vi "Set TimeToPlot.vi"(8 "error in (no error)":errorcluster, 10 "Time to Plot":dbl=1800.0 format="%<%H:%M:%S>t", 11 "Loop data in":T1 {"PanelMap"."Data"."Plot Bounds (%)"."Bottom (%)" format="%.2f"; "PanelMap"."Data"."Plot Bounds (%)"."Top (%)" format="%.2f"; "PanelMap"."Data"."Plot Bounds (%)"."Right (%)" format="%.2f"; "PanelMap"."Data"."Plot Bounds (%)"."Left (%)" format="%.2f"}) -> (0 "error out":errorcluster, 3 "Loop data out":T1 {"PanelMap"."Data"."Plot Bounds (%)"."Bottom (%)" format="%.2f"; "PanelMap"."Data"."Plot Bounds (%)"."Top (%)" format="%.2f"; "PanelMap"."Data"."Plot Bounds (%)"."Right (%)" format="%.2f"; "PanelMap"."Data"."Plot Bounds (%)"."Left (%)" format="%.2f"})   [LabVIEW 2021, in "MultiRocketPlotPanel.lvclass"]
uses:
  Classes/MultiPlotPanel/MultiRocketPlotPanel.lvclass
  Loop Data.ctl
  <vilib>/IlluminatedG/IG OOPanel/OOPanel/Manager/Manager.lvclass
  Panel Map.ctl
  Panel Map Data.ctl
  <userlib>/bjustice/RocketPlot/Classes/RocketPlotPanel/RocketPlotPanel.lvclass
  Window Position.ctl
  <vilib>/IlluminatedG/IG OOPanel/OOPanel/Panel/Panel Events.ctl
  <vilib>/IlluminatedG/IG OOPanel/OOPanel/Panel/Visbility Event Data.ctl
  <vilib>/IlluminatedG/IG OOPanel/OOPanel/Visibility State.ctl
  <vilib>/IlluminatedG/IG OOPanel/OOPanel/Close Reason.ctl
  <userlib>/bjustice/RocketPlot/Classes/RocketPlotPanel/RocketPlotPanel.lvclass/RocketPlotPanel.ctl
  <userlib>/bjustice/RocketPlot/Classes/RocketPlotPanel/Read RocketPlotHandle.vi
  <userlib>/bjustice/RocketPlot/Classes/RocketPlotHandle/RocketPlotHandle.lvclass
  <vilib>/IlluminatedG/IG OOPanel/OOPanel/OOPanel.lvlib
  <vilib>/IlluminatedG/IG OOPanel/OOPanel/Panel/Panel.lvclass
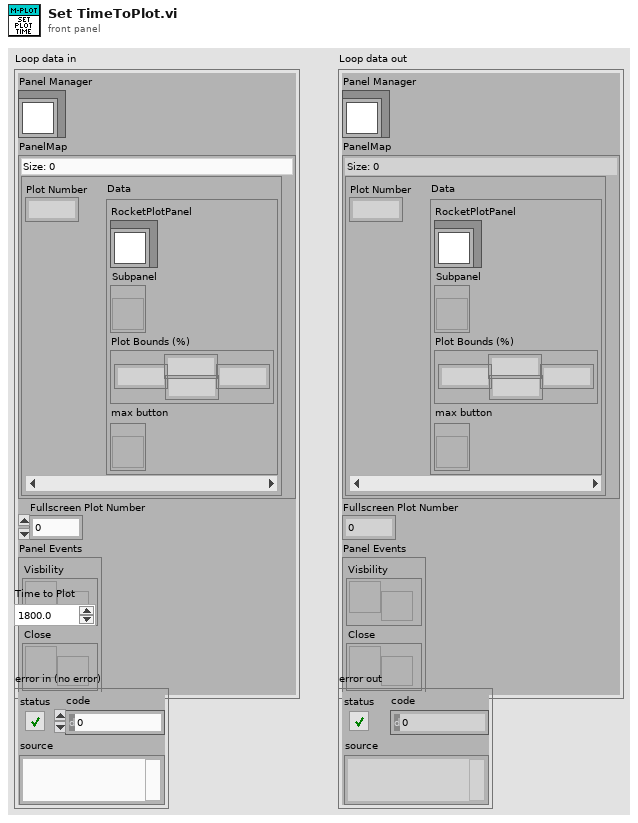
[diagram p1: front panel]
types:
  T1 = typedef "MultiRocketPlotPanel.lvclass/Loop Data.ctl" = cluster{"Panel Manager":refnum<class "Manager.lvclass">, "PanelMap":T2, "Fullscreen Plot Number":i32, "Panel Events":T5}
  T2 = typedef "MultiRocketPlotPanel.lvclass/Panel Map.ctl" = map{i32, T3}
  T3 = typedef "MultiRocketPlotPanel.lvclass/Panel Map Data.ctl" = cluster{"RocketPlotPanel":refnum<class "RocketPlotPanel.lvclass">, "Subpanel":refnum<vi>, "Plot Bounds (%)":T4, "max button":refnum<vi>}
  T4 = typedef "MultiRocketPlotPanel.lvclass/Window Position.ctl" = cluster{"Left (%)":dbl, "Top (%)":dbl, "Right (%)":dbl, "Bottom (%)":dbl}
  T5 = typedef "OOPanel.lvlib/Panel.lvclass/Panel Events.ctl" = cluster{"Visbility":refnum<user-event>, "Close":refnum<user-event>}
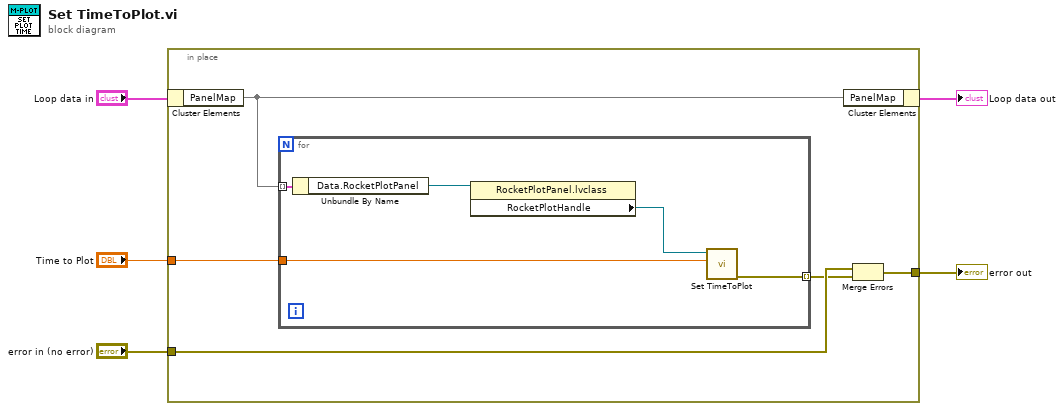
[diagram p0: block diagram]
diagram:
  n1 = in-place {
    in-place-border: "error in (no error)" -> [w9]
    in-place-border: [w6] -> w2
    in-place-border: "Time to Plot" -> [w7]
    n2 = in-place-cluster #1("Loop data in") -> ("PanelMap"=w10:T2)
    n3 = for {
      tunnel: w10 -> [w15] mode=indexing
      tunnel: [w11] -> w8 mode=indexing
      tunnel: w7 -> [w12]
      n4 = Unbundle By Name(w15) -> ("Data.RocketPlotPanel"=w14:refnum<class "RocketPlotPanel.lvclass">)
      n5 = property class="RocketPlotPanel.lvclass"(reference=w14) -> ("RocketPlotHandle"=w13:refnum<class "RocketPlotHandle.lvclass">)  [unwired: 1 in, 2 out]
      n6 = call <userlib>:"Set TimeToPlot.vi"("Time to Plot"=w12, "BluePlotHandle in"=w13) -> ("error out"=w11:errorcluster)  [unwired: 8 in, 1 out]
    }
    n7 = in-place-cluster #1("PanelMap"=w10) -> (→"Loop data out":T1)
    n8 = Merge Errors(w9, w8) -> (w6:errorcluster)
  }
  "error out" <- w2
